vi "VisualizeBase.vi"() -> ()   [LabVIEW 2017, in "Visualization.lvlib" / "VisualizeBase_class.lvclass"]
uses:
  VisualizeBase_class.lvclass
  Framework/Bus_class/Bus.lvclass
  Typedefs/VisualizeData.ctl
  Typedefs/clVisualizeData.ctl
  Modules/EventPlugins/EventPluginBaseClass/TypeDefs/clEvtReportArray.ctl
  Modules/EventPlugins/EventPluginBaseClass/TypeDefs/clEvtReport.ctl
  Modules/EventPlugins/EventPluginBaseClass/TypeDefs/dblEvtSignalArray.ctl
  Modules/NetworkImpairmentModule/PublicAPI/Arguments/Broadcasts/dblNetworkTime.ctl
  Modules/NetworkImpairmentModule/PublicAPI/Arguments/Broadcasts/dblPktLoss.ctl
  Modules/FlagImpairModule/PublicAPI/Arguments/Broadcasts/ui32FlagImpairmentArray.ctl
  Framework/Bus_class/Broadcast/Typedefs/clDidInit.ctl
  QMH/Typedefs/clEvtRptArray.ctl
  QMH/Typedefs/clEvtRptSignal.ctl
  QMH/Typedefs/clPmuImpairRptArray.ctl
  QMH/Typedefs/clNetImpairmentTime.ctl
  QMH/Typedefs/clNetIPktLoss.ctl
  QMH/Typedefs/clFlagImpairArray.ctl
  Requests/clUserEventType.ctl
  <vilib>/event_ctls.llb/usereventprio.ctl
  <vilib>/Utility/miscctls.llb/LVStringsAndValuesArrayTypeDef_U8.ctl
  <vilib>/Utility/error.llb/Error Cluster From Error Code.vi
  <vilib>/ErrorRing/Error Ring.xnode
  <userlib>/NIST/NISTErrorLib/NISTErrorLib.lvlib
  Framework/Bus_class/Bus_class.lvlib
  Modules/EventModule/EventModule.lvlib
  Modules/PmuImpairModule/PmuImpairModule.lvlib
  Modules/NetworkImpairmentModule/NetworkImpairmentModule.lvlib
  Modules/FlagImpairModule/FlagImpairModule.lvlib
  Modules/EventPlugins/EventPluginBaseClass/EventPluginBaseClass.lvclass
  VisualizeApp_class/VisualizeAppBase_class.lvclass
panel:
  in  "QueName":string="BaseVisQue"
  in  "Bus Number":u8(ring) items=[""=0, "2"=2]
  out "ErrorArray":errorcluster[](array[cluster])
  in  "btnStop":bool
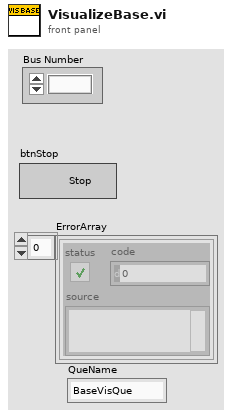
[diagram p1: front panel]
types:
  T1 = typedef "Visualization.lvlib/VisualizeBase_class.lvclass/VisualizeData.ctl" = T2[]
  T2 = typedef "Visualization.lvlib/VisualizeAppBase_class.lvclass/clVisualizeData.ctl" = cluster{"clEvtReportArray":T3, "dblEventSignalArray":T5, "clPmuImpairRptArray":T3, "dblNetworkTime":T6, "dblPktLoss":T7, "FlagImpairArray":T8, "TimeArray":dbl[]}
  T3 = typedef "EventPlugins.lvlib/EventPluginBaseClass.lvclass/clEvtReportArray.ctl" = T4[]
  T4 = typedef "EventPlugins.lvlib/EventPluginBaseClass.lvclass/clEvtReport.ctl" = cluster{"Timestamp":dbl, "Synx":cdb[], "Freq":dbl, "ROCOF":dbl, "ID":i16}
  T5 = typedef "EventPlugins.lvlib/EventPluginBaseClass.lvclass/dblEvtSignalArray.ctl" = dbl[][]
  T6 = typedef "NetworkImpairmentModule.lvlib/dblNetworkTime.ctl" = dbl[]
  T7 = typedef "NetworkImpairmentModule.lvlib/dblPktLoss.ctl" = dbl[]
  T8 = typedef "FlagImpairModule.lvlib/ui32FlagImpairmentArray.ctl" = u32[]
  T9 = typedef "Visualization.lvlib/VisualizeBase_class.lvclass/clRequestEvents.ctl" = cluster{"StopRequest":refnum<user-event>}
  T10 = typedef "Bus_class.lvlib/clBroadcastEvents.ctl" = cluster{"DidInit":refnum<user-event>, "DidStop":refnum<user-event>}
  T11 = typedef "EventModule.lvlib/clBroadcastEvents.ctl" = cluster{"DidInit":refnum<user-event>, "StatusUpdate":refnum<user-event>, "ErrorReport":refnum<user-event>, "DidStop":refnum<user-event>, "ReadEvtConfig":refnum<user-event>, "ReadTimeArray":refnum<user-event>, "ReadEvtParams":refnum<user-event>, "GetEvtReportArray":refnum<user-event>, "ReadPathToPlugin":refnum<user-event>, "GetEvtSignal":refnum<user-event>, "ReadBusNumber":refnum<user-event>}
  T12 = typedef "PmuImpairModule.lvlib/clBroadcastEvents.ctl" = cluster{"DidInit":refnum<user-event>, "StatusUpdate":refnum<user-event>, "ErrorReport":refnum<user-event>, "DidStop":refnum<user-event>, "ImpairConfig":refnum<user-event>, "ImpairParams":refnum<user-event>, "ImpairReports":refnum<user-event>, "PathToPlugin":refnum<user-event>, "BusNumber":refnum<user-event>}
  T13 = typedef "NetworkImpairmentModule.lvlib/clBroadcastEvents.ctl" = cluster{"DidInit":refnum<user-event>, "StatusUpdate":refnum<user-event>, "ErrorReport":refnum<user-event>, "DidStop":refnum<user-event>, "ReadNetImpParams":refnum<user-event>, "ReadLossThreshold":refnum<user-event>, "GetNetworkTime":refnum<user-event>, "GetPktLoss":refnum<user-event>, "ReadPathToPlugin":refnum<user-event>}
  T14 = typedef "FlagImpairModule.lvlib/clBroadcastEvents.ctl" = cluster{"DidInit":refnum<user-event>, "StatusUpdate":refnum<user-event>, "ErrorReport":refnum<user-event>, "DidStop":refnum<user-event>, "ReadFlagImpairConfig":refnum<user-event>, "ReadPluginINIFilePath":refnum<user-event>, "ReadFlagImpairParams":refnum<user-event>, "ReadTimeArray":refnum<user-event>, "GetFlagImpairment":refnum<user-event>}
  T15 = typedef "LVStringsAndValuesArrayTypeDef_U8.ctl" = cluster{"String":string, "Value":u8}[]
  T16 = typedef "Visualization.lvlib/VisualizeBase_class.lvclass/clEvtRptArray.ctl" = cluster{"BusIndex":i32, "clImpairReportArray":T3}
  T17 = typedef "Visualization.lvlib/VisualizeBase_class.lvclass/clPmuImpairRptArray.ctl" = cluster{"BusIndex":i32, "clImpairReportArray":T3}
  T18 = typedef "Visualization.lvlib/VisualizeBase_class.lvclass/clNetImpairmentTime.ctl" = cluster{"BusIndex":i32, "clNetImpairTimeArray":T6}
  T19 = typedef "Visualization.lvlib/VisualizeBase_class.lvclass/clNetIPktLoss.ctl" = cluster{"BusIndex":i32, "clNetPktLoss":T7}
  T20 = typedef "Visualization.lvlib/VisualizeBase_class.lvclass/clFlagImpairArray.ctl" = cluster{"BusIndex":i32, "FlagImpairArray":T8}
  T21 = typedef "Visualization.lvlib/VisualizeBase_class.lvclass/clEvtRptSignal.ctl" = cluster{"BusIndex":i32, "dblEventSignalArray":T5}
  T22 = typedef "Visualization.lvlib/VisualizeBase_class.lvclass/clUserEventType.ctl" = cluster{"BusIndex":i8, "Data":variant}
  T23 = typedef "usereventprio.ctl" = enum32{"high priority", "normal priority"}
  T24 = typedef "Bus_class.lvlib/clDidInit.ctl" = cluster{"Bus":refnum<vi>, "Init?":bool}
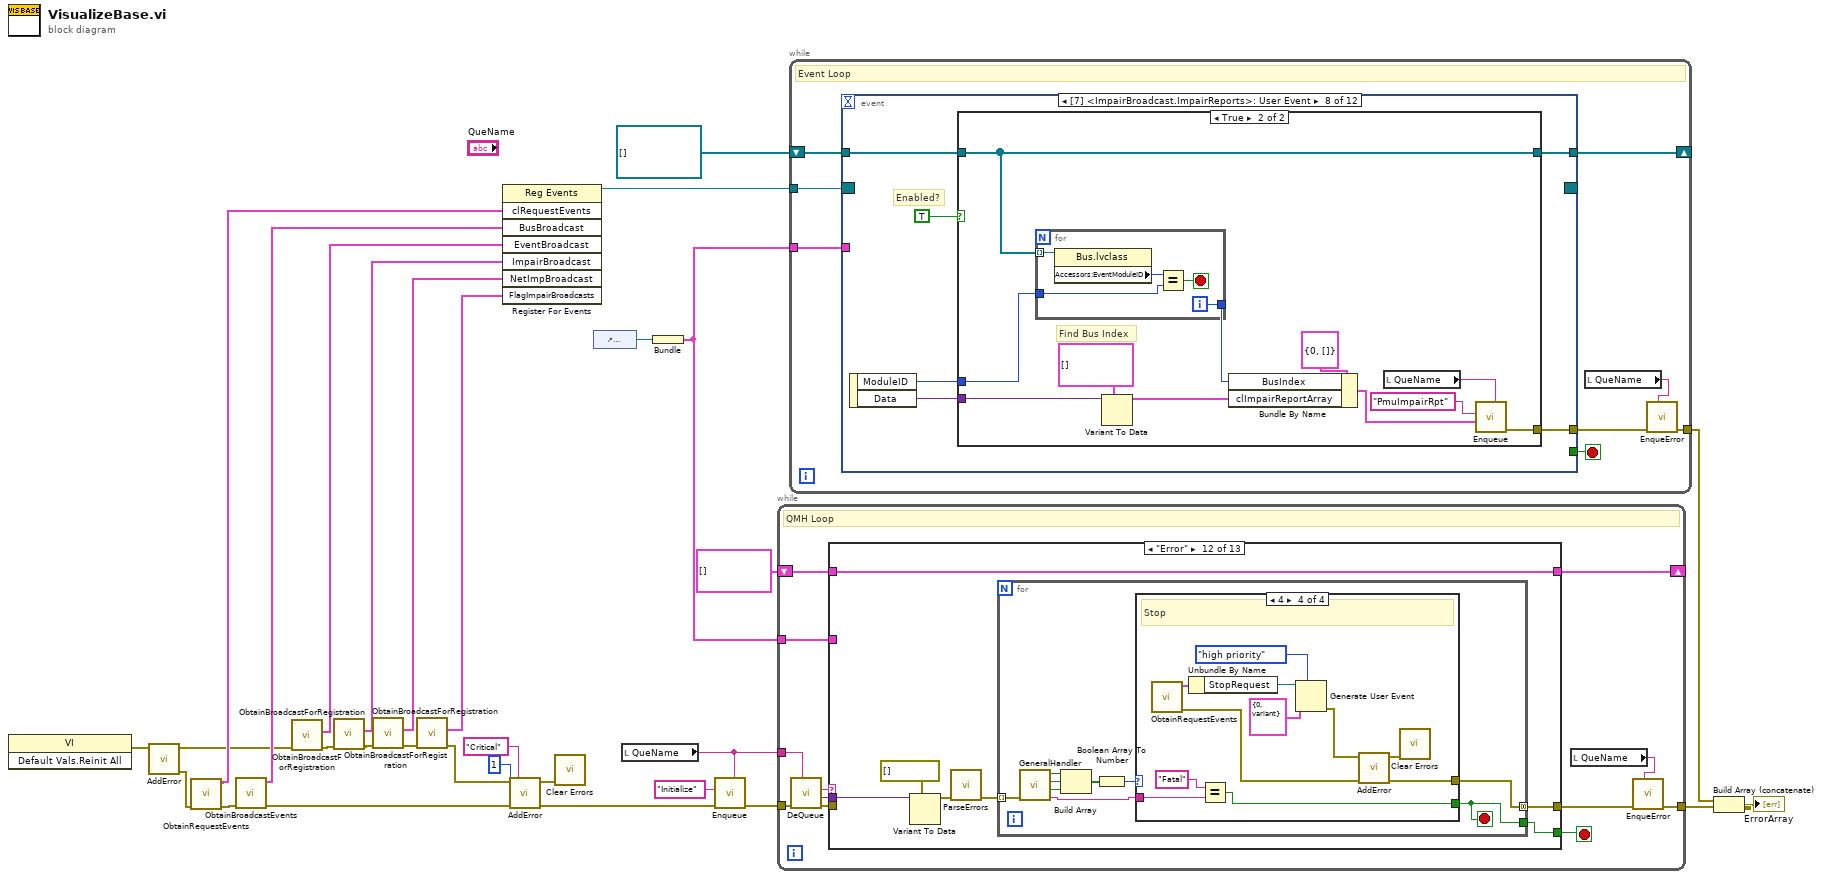
[diagram p0: block diagram]
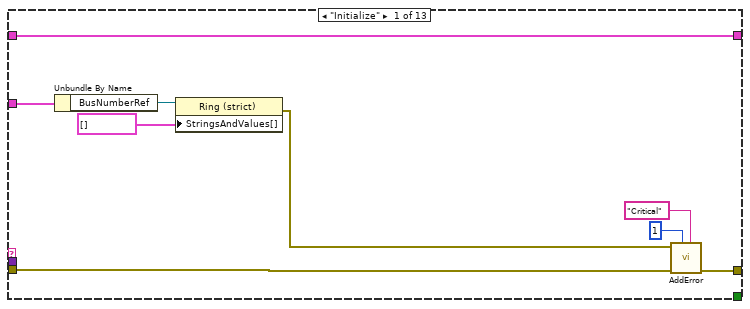
[diagram p2: hidden frame]
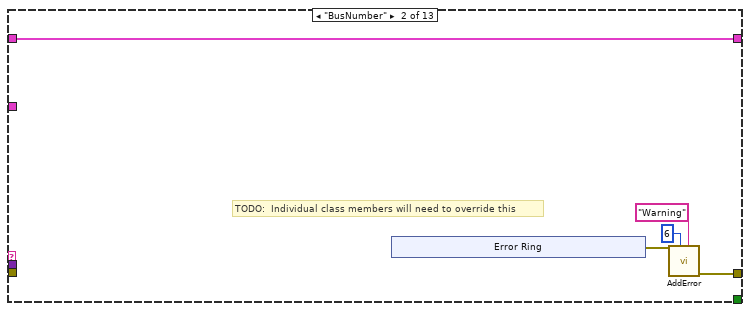
[diagram p3: hidden frame]
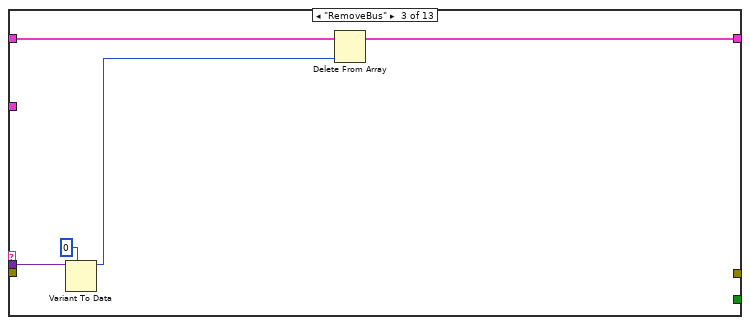
[diagram p4: hidden frame]
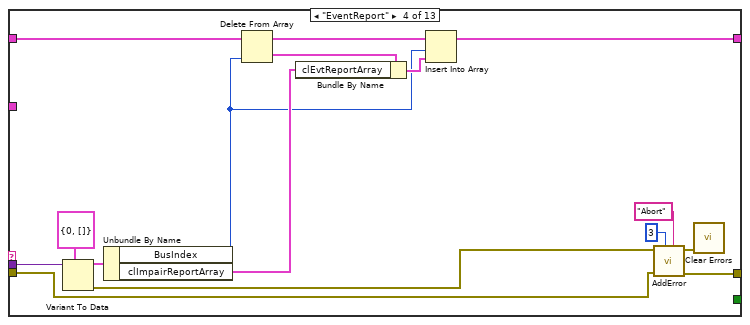
[diagram p5: hidden frame]
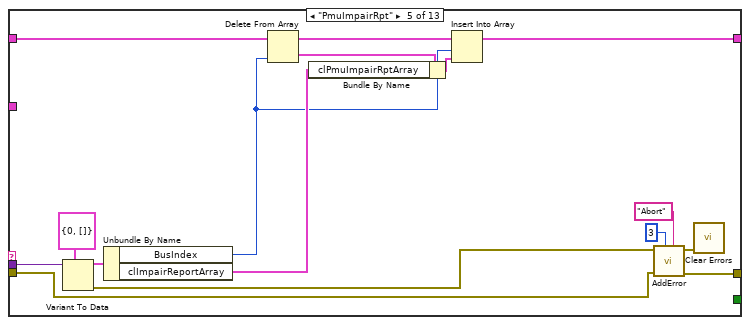
[diagram p6: hidden frame]
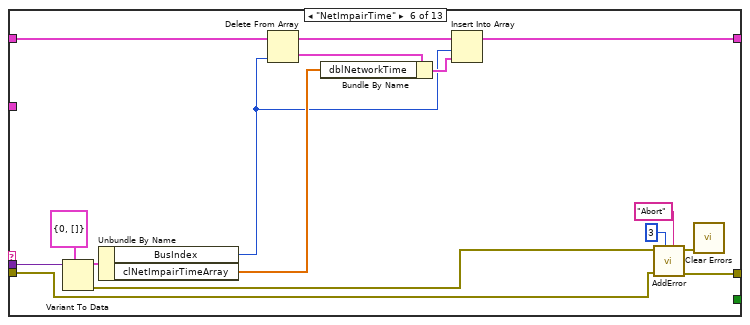
[diagram p7: hidden frame]
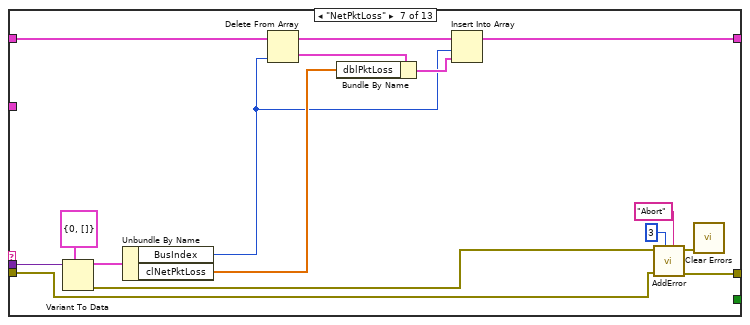
[diagram p8: hidden frame]
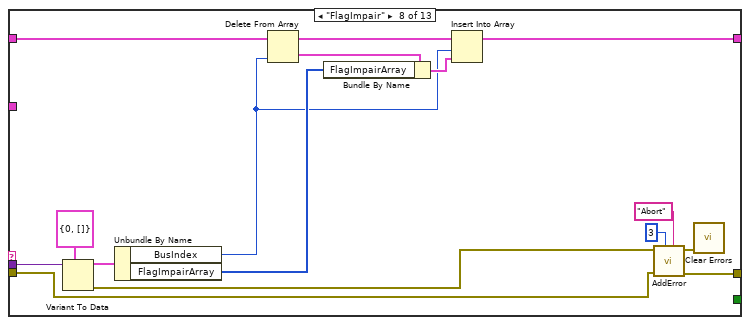
[diagram p9: hidden frame]
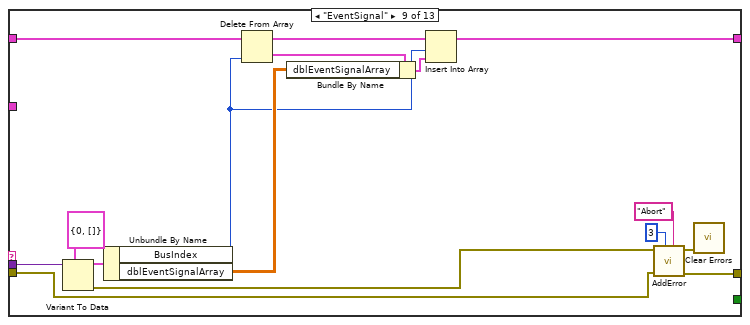
[diagram p10: hidden frame]
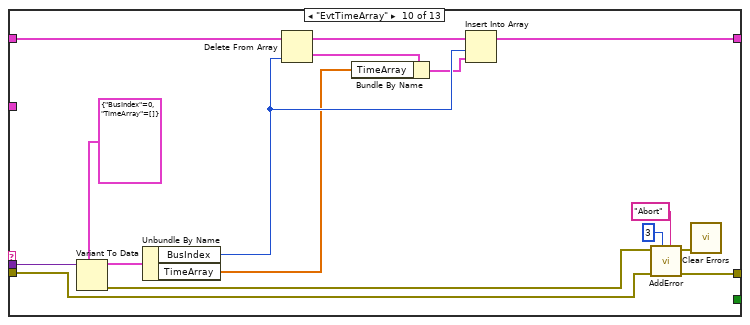
[diagram p11: hidden frame]
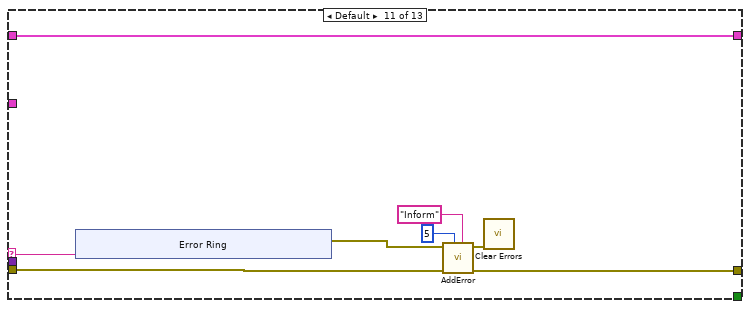
[diagram p12: hidden frame]
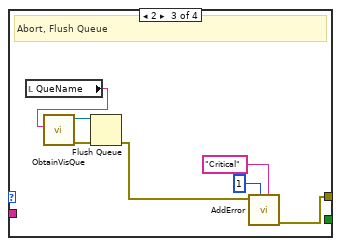
[diagram p15: hidden frame]
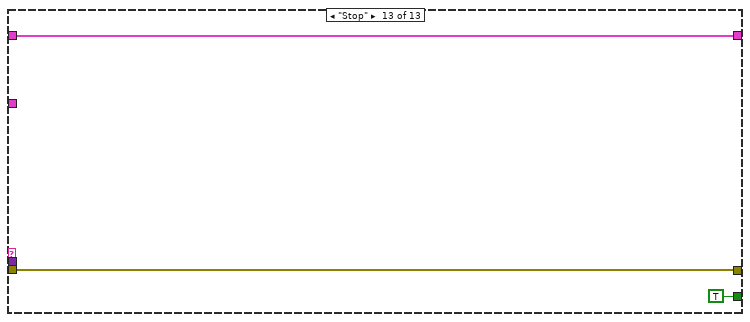
[diagram p16: hidden frame]
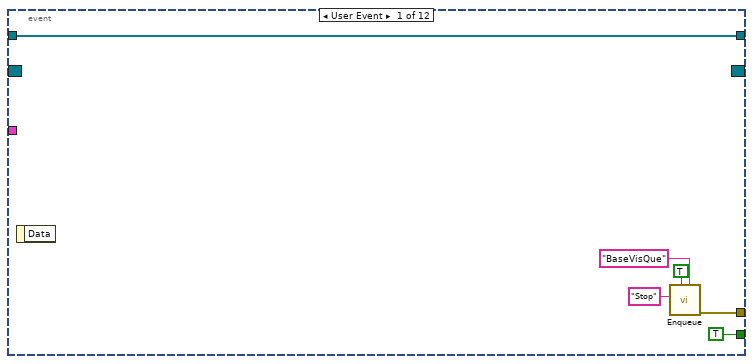
[diagram p17: hidden frame]
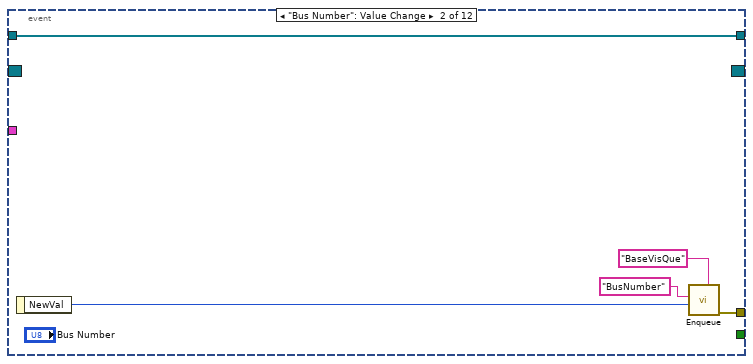
[diagram p18: hidden frame]
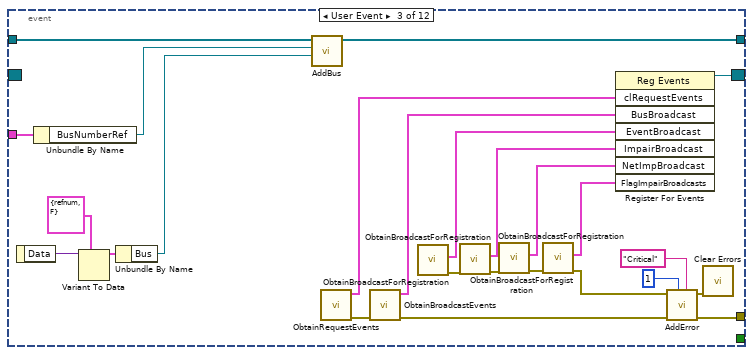
[diagram p19: hidden frame]
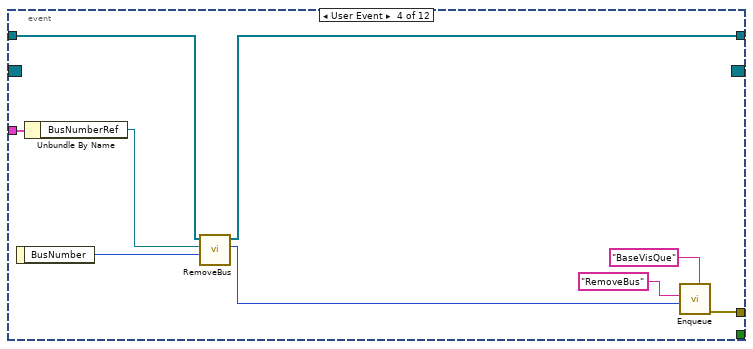
[diagram p20: hidden frame]
diagram:
  n1 = invoke class="VI" method="Default Vals.Reinit All"() -> (error out=w19:errorcluster)  [unwired: 3 in, 2 out]
  n2 = call <userlib>:"AddError.vi"("error in (no error)"=w19) -> ("ErrorArray"=w18:errorcluster[], "error out"=w10:errorcluster)  [unwired: 9 in]
  n3 = call "ObtainRequestEvents.vi"("Error"=w18) -> ("Error"=w23:errorcluster[], "clRequestEvents"=w28:T9)  [unwired: 9 in]
  n4 = call "ObtainBroadcastEvents.vi"("ErrorArray"=w23) -> ("ErrorArray"=w9:errorcluster[], "BusBroadcast"=w22:T10)  [unwired: 9 in]
  n5 = call "ObtainBroadcastForRegistration.vi"("error in (no error)"=w10) -> ("error out"=w13:errorcluster, "EventBroadcast"=w17:T11)  [unwired: 9 in]
  n6 = call "ObtainBroadcastForRegistration.vi"("error in (no error)"=w13) -> ("error out"=w12:errorcluster, "ImpairBroadcast"=w16:T12)  [unwired: 9 in]
  n7 = call "ObtainBroadcastForRegistration.vi"("error in (no error)"=w12) -> ("error out"=w11:errorcluster, "NetImpBroadcast"=w15:T13)  [unwired: 9 in]
  n8 = call "ObtainBroadcastForRegistration.vi"("error in (no error)"=w11) -> ("error out"=w8:errorcluster, "FlagImpairBroadcasts"=w14:T14)  [unwired: 9 in]
  n9 = register-events(w28, w22, w17, w16, w15, w14) -> (reference out=w27:refnum<event-registration>)  [unwired: 2 in, 1 out]
  n10 = call <userlib>:"AddError.vi"("Severity"="Critical" ("String"), "Priority"=u8 1, "ErrorArray"=w9, "error in (no error)"=w8) -> ("ErrorArray"=w5:errorcluster[], "error out"=w2:errorcluster)  [unwired: 6 in]
  n11 = call <vilib>:"Clear Errors.vi"("error in (no error)"=w2) -> ()  [unwired: 5 in, 2 out]
  n12 = control-ref of="BusNumberRef"() -> (w21:refnum<vi>)
  n13 = local read "QueName"() -> (w1:string)
  n14 = Bundle("BusNumberRef"=w21) -> (w3:cluster{"BusNumberRef":refnum<vi>})  [unwired: 1 in]
  n15 = call "Enqueue.vi"("QueName"=w1, "Error"=w5, "Message"="Initialize") -> ("Error"=w29:errorcluster[])  [unwired: 8 in]
  n16 = while {
    tunnel: w29 -> [w42]
    tunnel: [w36] -> w26
    tunnel: w3 -> [w35]
    shift-right: [w33] -> _
    shift-left: T1 [] ("VisualizeData") -> [w34]
    tunnel: w1 -> [w31]
    stop <- w37 stop-if-true
    # "QMH Loop"
    n17 = call "DeQueue.vi"("QueName"=w31, "Error"=w42) -> ("Error"=w39:errorcluster[], "Data"=w40:variant, "Message"=w41:string)  [unwired: 7 in]
    n18 = case shown="\"Error\"" w41 {
      selector: w41 -> [_ _ _ _ _ _ _ _ _ _ w186 _ _]
      tunnel: w40 -> [_ _ w66 w82 w98 w114 w130 w146 w162 w169 _ w200 _]
      tunnel: w39 -> [w48 _ _ w67 w83 w99 w115 w131 w147 w163 w184 _ w229]
      tunnel: [w47 w56 _ w72 w88 w104 w120 w136 w152 w165 w183 w196 w229] -> w38
      tunnel: [_ _ _ _ _ _ _ _ _ _ _ w195 TRUE] -> w37
      tunnel: w35 -> [w51 _ _ _ _ _ _ _ _ _ _ _ _]
      tunnel: w34 -> [w43 w52 w64 w78 w94 w110 w126 w142 w158 w171 w179 w194 w228]
      tunnel: [w43 w52 w63 w79 w95 w111 w127 w143 w159 w170 w179 w194 w228] -> w33
      frame "Initialize" {
        n19 = Unbundle By Name(w51) -> ("BusNumberRef"=w50:refnum<vi>)
        n20 = property class="Ring (strict)"(reference=w50, "StringsAndValues[]"=T15 [] ("Strings And Values []")) -> (error out=w46:errorcluster)  [unwired: 1 in, 1 out]
        n21 = call <userlib>:"AddError.vi"("Severity"="Critical" ("String"), "Priority"=u8 1, "ErrorArray"=w48, "error in (no error)"=w46) -> ("ErrorArray"=w47:errorcluster[])  [unwired: 6 in, 1 out]
      }
      frame "BusNumber" {
        # "TODO:  Individual class members will need to override this"
        n22 = xnode "Error Ring"() -> ("error out"=w55:errorcluster)
        n23 = call <userlib>:"AddError.vi"("Severity"="Warning" ("String"), "Priority"=u8 6, "error in (no error)"=w55) -> ("ErrorArray"=w56:errorcluster[])  [unwired: 7 in, 1 out]
      }
      frame "RemoveBus" {
        n24 = Variant To Data(type=0, Variant=w66) -> (data=w62:i32)  [unwired: 1 in, 1 out]
        n25 = Delete From Array(array=w64, index=w62) -> (array with subset deleted=w63:T1)  [unwired: 1 in, 1 out]
      }
      frame "EventReport" {
        n26 = Variant To Data(type=T16 {"BusIndex"=0, "clImpairReportArray"=[]} ("clEvtReportArray"), Variant=w82) -> (data=w80:T16, error out=w71:errorcluster)  [unwired: 1 in]
        n27 = Unbundle By Name(w80) -> ("BusIndex"=w73:i32, "clImpairReportArray"=w75:T3)
        n28 = Delete From Array(array=w78, index=w73) -> (deleted portion=w76:T2, array with subset deleted=w77:T1)  [unwired: 1 in]
        n29 = Bundle By Name(cluster=w76, "clEvtReportArray"=w75) -> (w74:T2)
        n30 = Insert Into Array(array=w77, index=w73, new element=w74) -> (w79:T1)
        n31 = call <userlib>:"AddError.vi"("Severity"="Abort" ("String"), "Priority"=u8 3, "ErrorArray"=w67, "error in (no error)"=w71) -> ("ErrorArray"=w72:errorcluster[], "error out"=w70:errorcluster)  [unwired: 6 in]
        n32 = call <vilib>:"Clear Errors.vi"("error in (no error)"=w70) -> ()  [unwired: 5 in, 2 out]
      }
      frame "PmuImpairRpt" {
        n33 = Variant To Data(type=T17 {"BusIndex"=0, "clImpairReportArray"=[]} ("clImpairReportArray"), Variant=w98) -> (data=w96:T17, error out=w87:errorcluster)  [unwired: 1 in]
        n34 = Unbundle By Name(w96) -> ("BusIndex"=w89:i32, "clImpairReportArray"=w91:T3)
        n35 = Delete From Array(array=w94, index=w89) -> (deleted portion=w92:T2, array with subset deleted=w93:T1)  [unwired: 1 in]
        n36 = Bundle By Name(cluster=w92, "clPmuImpairRptArray"=w91) -> (w90:T2)
        n37 = Insert Into Array(array=w93, index=w89, new element=w90) -> (w95:T1)
        n38 = call <userlib>:"AddError.vi"("Severity"="Abort" ("String"), "Priority"=u8 3, "ErrorArray"=w83, "error in (no error)"=w87) -> ("ErrorArray"=w88:errorcluster[], "error out"=w86:errorcluster)  [unwired: 6 in]
        n39 = call <vilib>:"Clear Errors.vi"("error in (no error)"=w86) -> ()  [unwired: 5 in, 2 out]
      }
      frame "NetImpairTime" {
        n40 = Variant To Data(type=T18 {"BusIndex"=0, "clNetImpairTimeArray"=[]} ("clImpairReportArray"), Variant=w114) -> (data=w112:T18, error out=w103:errorcluster)  [unwired: 1 in]
        n41 = Unbundle By Name(w112) -> ("BusIndex"=w105:i32, "clNetImpairTimeArray"=w107:T6)
        n42 = Delete From Array(array=w110, index=w105) -> (deleted portion=w108:T2, array with subset deleted=w109:T1)  [unwired: 1 in]
        n43 = Bundle By Name(cluster=w108, "dblNetworkTime"=w107) -> (w106:T2)
        n44 = Insert Into Array(array=w109, index=w105, new element=w106) -> (w111:T1)
        n45 = call <userlib>:"AddError.vi"("Severity"="Abort" ("String"), "Priority"=u8 3, "ErrorArray"=w99, "error in (no error)"=w103) -> ("ErrorArray"=w104:errorcluster[], "error out"=w102:errorcluster)  [unwired: 6 in]
        n46 = call <vilib>:"Clear Errors.vi"("error in (no error)"=w102) -> ()  [unwired: 5 in, 2 out]
      }
      frame "NetPktLoss" {
        n47 = Variant To Data(type=T19 {"BusIndex"=0, "clNetPktLoss"=[]} ("clNetPktLoss"), Variant=w130) -> (data=w128:T19, error out=w119:errorcluster)  [unwired: 1 in]
        n48 = Unbundle By Name(w128) -> ("BusIndex"=w121:i32, "clNetPktLoss"=w123:T7)
        n49 = Delete From Array(array=w126, index=w121) -> (deleted portion=w124:T2, array with subset deleted=w125:T1)  [unwired: 1 in]
        n50 = Bundle By Name(cluster=w124, "dblPktLoss"=w123) -> (w122:T2)
        n51 = Insert Into Array(array=w125, index=w121, new element=w122) -> (w127:T1)
        n52 = call <userlib>:"AddError.vi"("Severity"="Abort" ("String"), "Priority"=u8 3, "ErrorArray"=w115, "error in (no error)"=w119) -> ("ErrorArray"=w120:errorcluster[], "error out"=w118:errorcluster)  [unwired: 6 in]
        n53 = call <vilib>:"Clear Errors.vi"("error in (no error)"=w118) -> ()  [unwired: 5 in, 2 out]
      }
      frame "FlagImpair" {
        n54 = Variant To Data(type=T20 {"BusIndex"=0, "FlagImpairArray"=[]} ("clFlagImpairArray"), Variant=w146) -> (data=w144:T20, error out=w135:errorcluster)  [unwired: 1 in]
        n55 = Unbundle By Name(w144) -> ("BusIndex"=w137:i32, "FlagImpairArray"=w139:T8)
        n56 = Delete From Array(array=w142, index=w137) -> (deleted portion=w140:T2, array with subset deleted=w141:T1)  [unwired: 1 in]
        n57 = Bundle By Name(cluster=w140, "FlagImpairArray"=w139) -> (w138:T2)
        n58 = Insert Into Array(array=w141, index=w137, new element=w138) -> (w143:T1)
        n59 = call <userlib>:"AddError.vi"("Severity"="Abort" ("String"), "Priority"=u8 3, "ErrorArray"=w131, "error in (no error)"=w135) -> ("ErrorArray"=w136:errorcluster[], "error out"=w134:errorcluster)  [unwired: 6 in]
        n60 = call <vilib>:"Clear Errors.vi"("error in (no error)"=w134) -> ()  [unwired: 5 in, 2 out]
      }
      frame "EventSignal" {
        n61 = Variant To Data(type=T21 {"BusIndex"=0, "dblEventSignalArray"=[]} ("clEvtReportArray"), Variant=w162) -> (data=w160:T21, error out=w151:errorcluster)  [unwired: 1 in]
        n62 = Unbundle By Name(w160) -> ("BusIndex"=w153:i32, "dblEventSignalArray"=w155:T5)
        n63 = Delete From Array(array=w158, index=w153) -> (deleted portion=w156:T2, array with subset deleted=w157:T1)  [unwired: 1 in]
        n64 = Bundle By Name(cluster=w156, "dblEventSignalArray"=w155) -> (w154:T2)
        n65 = Insert Into Array(array=w157, index=w153, new element=w154) -> (w159:T1)
        n66 = call <userlib>:"AddError.vi"("Severity"="Abort" ("String"), "Priority"=u8 3, "ErrorArray"=w147, "error in (no error)"=w151) -> ("ErrorArray"=w152:errorcluster[], "error out"=w150:errorcluster)  [unwired: 6 in]
        n67 = call <vilib>:"Clear Errors.vi"("error in (no error)"=w150) -> ()  [unwired: 5 in, 2 out]
      }
      frame "EvtTimeArray" {
        n68 = Variant To Data(type=cluster{"BusIndex":i32, "TimeArray":dbl[]} {"BusIndex"=0, "TimeArray"=[]} ("cluster"), Variant=w169) -> (data=w172:cluster{"BusIndex":i32, "TimeArray":dbl[]}, error out=w164:errorcluster)  [unwired: 1 in]
        n69 = Unbundle By Name(w172) -> ("BusIndex"=w177:i32, "TimeArray"=w175:dbl[])
        n70 = Delete From Array(array=w171, index=w177) -> (deleted portion=w174:T2, array with subset deleted=w173:T1)  [unwired: 1 in]
        n71 = Bundle By Name(cluster=w174, "TimeArray"=w175) -> (w176:T2)
        n72 = Insert Into Array(array=w173, index=w177, new element=w176) -> (w170:T1)
        n73 = call <userlib>:"AddError.vi"("Severity"="Abort" ("String"), "Priority"=u8 3, "ErrorArray"=w163, "error in (no error)"=w164) -> ("ErrorArray"=w165:errorcluster[], "error out"=w166:errorcluster)  [unwired: 6 in]
        n74 = call <vilib>:"Clear Errors.vi"("error in (no error)"=w166) -> ()  [unwired: 5 in, 2 out]
      }
      frame Default {
        n75 = xnode "Error Ring"("parameter 0"=w186) -> ("error out"=w185:errorcluster)
        n76 = call <userlib>:"AddError.vi"("Severity"="Inform" ("String"), "Priority"=u8 5, "ErrorArray"=w184, "error in (no error)"=w185) -> ("ErrorArray"=w183:errorcluster[], "error out"=w182:errorcluster)  [unwired: 6 in]
        n77 = call <vilib>:"Clear Errors.vi"("error in (no error)"=w182) -> ()  [unwired: 5 in, 2 out]
      }
      frame "Error" {
        n78 = Variant To Data(type=errorcluster[] [], Variant=w200) -> (data=w198:errorcluster[])  [unwired: 1 in, 1 out]
        n79 = call <userlib>:"ParseErrors.vi"("ErrorArray"=w198) -> ("ErrorArray"=w197:errorcluster[])  [unwired: 8 in, 2 out]
        n80 = for {
          tunnel: w197 -> [w209] mode=indexing
          tunnel: [w203] -> w196 mode=concatenating
          tunnel: [w201] -> w195
          stop <- w201 stop-if-true
          n81 = call <userlib>:"GeneralHandler.vi"("error in (no error)"=w209) -> ("Severity"=w202:string, "Stop"=w206:bool, "Abort"=w207:bool, "Continue"=w208:bool)  [unwired: 7 in]
          n82 = Build Array(w208, w207, w206) -> (w205:bool[])
          n83 = Boolean Array To Number(Boolean array=w205) -> (number=w204:u32)
          n84 = case shown="4" w204 {
            tunnel: [_ _ w214 w225] -> w203
            tunnel: w202 -> [_ _ _ w219]
            tunnel: [_ _ _ w217] -> w201
            frame 0, Default {
              # "No Dialog"
            }
            frame 1 {
              # "Continue"
            }
            frame 2 {
              # "Abort, Flush Queue"
              n85 = local read "QueName"() -> (w210:string)
              n86 = call "ObtainVisQue.vi"("QueName"=w210) -> ("error out"=w216:errorcluster, "queue out"=w215:refnum<queue>)  [unwired: 9 in]
              n87 = Flush Queue(queue=w215, error in (no error)=w216) -> (error out=w213:errorcluster)  [unwired: 2 out]
              n88 = call <userlib>:"AddError.vi"("Severity"="Critical" ("String"), "Priority"=u8 1, "error in (no error)"=w213) -> ("ErrorArray"=w214:errorcluster[])  [unwired: 7 in, 1 out]
            }
            frame 4 {
              # "Stop"
              n89 = call "ObtainRequestEvents.vi"() -> ("Error"=w223:errorcluster[], "clRequestEvents"=w227:T9)  [unwired: 10 in]
              n90 = Unbundle By Name(w227) -> ("StopRequest"=w226:refnum<user-event>)
              n91 = Equal?(x="Fatal", y=w219) -> (x = y?=w217:bool)
              n92 = Generate User Event(priority (normal)=usereventprio."high priority", user event=w226, event data cluster=T22 {"BusIndex"=0, "Data"=variant} ("event data")) -> (error out=w224:errorcluster)  [unwired: 1 in, 1 out]
              n93 = call <userlib>:"AddError.vi"("ErrorArray"=w223, "error in (no error)"=w224) -> ("ErrorArray"=w225:errorcluster[], "error out"=w220:errorcluster)  [unwired: 8 in]
              n94 = call <vilib>:"Clear Errors.vi"("error in (no error)"=w220) -> ()  [unwired: 5 in, 2 out]
            }
          }
        }
      }
      frame "Stop" {
      }
    }
    n95 = local read "QueName"() -> (w32:string)
    n96 = call "EnqueError.vi"("QueName"=w32, "Error"=w38) -> ("Error"=w36:errorcluster[])  [unwired: 9 in]
  }
  n97 = while {
    tunnel: w27 -> [w238]
    tunnel: [w235] -> w25
    tunnel: w3 -> [w234]
    shift-right: [w232] -> _
    shift-left: refnum<class "Bus.lvclass">[] [] -> [w233]
    stop <- w237 stop-if-true
    # "Event Loop"
    n98 = event shown="[7] <ImpairBroadcast.ImpairReports>: User Event" {
      selector: w238 -> [_ _ _ _ _ _ _ _ _ _ _ _]
      dyn-events: [_ _ w258 _ _ _ _ _ _ _ _ _] -> _
      timeout: _ -> [_ _ _ _ _ _ _ _ _ _ _ _]
      tunnel: [TRUE _ _ _ _ _ _ _ _ _ _ _] -> w237
      tunnel: [w243 w249 w261 w279 w285 w314 w337 w360 w383 w406 w429 w456] -> w236
      tunnel: w234 -> [_ _ w271 w283 _ _ _ _ _ _ _ _]
      tunnel: w233 -> [w240 w246 w270 w282 w286 w317 w340 w363 w386 w409 w432 w450]
      tunnel: [w240 w246 w267 w281 w284 w312 w335 w358 w381 w404 w427 w450] -> w232
      event User Event {
        n99 = event-data() -> ()  [unwired: 1 in, 1 out]
        n100 = call "Enqueue.vi"("QueName"="BaseVisQue", "Priority? (F)"=TRUE, "Message"="Stop") -> ("Error"=w243:errorcluster[])  [unwired: 8 in]
      }
      event "Bus Number": Value Change {
        n101 = event-data() -> ("NewVal"=w248:u8)  [unwired: 1 in]
        n102 = call "Enqueue.vi"("QueName"="BaseVisQue", "Data"=w248, "Message"="BusNumber") -> ("Error"=w249:errorcluster[])  [unwired: 8 in]
      }
      event User Event {
        n103 = event-data() -> ("Data"=w274:variant)  [unwired: 1 in]
        n104 = Unbundle By Name(w271) -> ("BusNumberRef"=w269:refnum<vi>)
        n105 = Variant To Data(type=T24 {"Bus"=refnum, "Init?"=FALSE} ("clBusDidInit"), Variant=w274) -> (data=w272:T24)  [unwired: 1 in, 1 out]
        n106 = Unbundle By Name(w272) -> ("Bus"=w268:refnum<vi>)
        n107 = call "AddBus.vi"("BusRef"=w268, "BusNumberRef"=w269, "BusArray"=w270) -> ("BusArray"=w267:refnum<class "Bus.lvclass">[])  [unwired: 8 in]
        n108 = call "ObtainRequestEvents.vi"() -> ("Error"=w253:errorcluster[], "clRequestEvents"=w251:T9)  [unwired: 10 in]
        n109 = call "ObtainBroadcastEvents.vi"("ErrorArray"=w253) -> ("ErrorArray"=w252:errorcluster[], "BusBroadcast"=w250:T10)  [unwired: 9 in]
        n110 = call "ObtainBroadcastForRegistration.vi"() -> ("error out"=w266:errorcluster, "EventBroadcast"=w257:T11)  [unwired: 10 in]
        n111 = call "ObtainBroadcastForRegistration.vi"("error in (no error)"=w266) -> ("error out"=w265:errorcluster, "ImpairBroadcast"=w256:T12)  [unwired: 9 in]
        n112 = call "ObtainBroadcastForRegistration.vi"("error in (no error)"=w265) -> ("error out"=w264:errorcluster, "NetImpBroadcast"=w255:T13)  [unwired: 9 in]
        n113 = call "ObtainBroadcastForRegistration.vi"("error in (no error)"=w264) -> ("error out"=w259:errorcluster, "FlagImpairBroadcasts"=w254:T14)  [unwired: 9 in]
        n114 = register-events(w251, w250, w257, w256, w255, w254) -> (reference out=w258:refnum<event-registration>)  [unwired: 2 in, 1 out]
        n115 = call <userlib>:"AddError.vi"("Severity"="Critical" ("String"), "Priority"=u8 1, "ErrorArray"=w252, "error in (no error)"=w259) -> ("ErrorArray"=w261:errorcluster[], "error out"=w260:errorcluster)  [unwired: 6 in]
        n116 = call <vilib>:"Clear Errors.vi"("error in (no error)"=w260) -> ()  [unwired: 5 in, 2 out]
      }
      event User Event {
        n117 = event-data() -> ("BusNumber"=w276:i8)  [unwired: 1 in]
        n118 = Unbundle By Name(w283) -> ("BusNumberRef"=w280:refnum<vi>)
        n119 = call "RemoveBus.vi"("BusArray"=w282, "BusNumberRef"=w280, "BusNumber"=w276) -> ("BusArray"=w281:refnum<class "Bus.lvclass">[], "BusIndex"=w278:i32)  [unwired: 6 in]
        n120 = call "Enqueue.vi"("QueName"="BaseVisQue", "Data"=w278, "Message"="RemoveBus") -> ("Error"=w279:errorcluster[])  [unwired: 8 in]
      }
      event User Event {
        w287 = TRUE  # Enabled?
        n121 = event-data() -> ("ModuleID"=w289:i32, "Data"=w288:variant)  [unwired: 1 in]
        n122 = case shown="True" w287 {
          tunnel: [w290 w306] -> w284
          tunnel: w286 -> [w290 w306]
          tunnel: w289 -> [_ w303]
          tunnel: w288 -> [_ w305]
          tunnel: [_ w293] -> w285
          frame False {
          }
          frame True {
            n123 = Variant To Data(type=dbl[] [], Variant=w305) -> (data=w302:dbl[], error out=w298:errorcluster)  [unwired: 1 in]
            n124 = for {
              tunnel: w306 -> [w311] mode=indexing
              tunnel: w303 -> [w309]
              tunnel: [w307] -> w292
              i -> [w307]
              stop <- w308 stop-if-true
              # "Find Bus Index"
              n125 = property class="Bus.lvclass"(reference=w311) -> ("Accessors:EventModuleID"=w310:i32)  [unwired: 1 in, 2 out]
              n126 = Equal?(x=w310, y=w309) -> (x = y?=w308:bool)
            }
            n127 = call <userlib>:"AddError.vi"("Severity"="Critical" ("String"), "Priority"=u8 1, "error in (no error)"=w298) -> ("ErrorArray"=w294:errorcluster[], "error out"=w297:errorcluster)  [unwired: 7 in]
            n128 = call <vilib>:"Clear Errors.vi"("error in (no error)"=w297) -> ()  [unwired: 5 in, 2 out]
            n129 = Bundle(w292, w302) -> (w301:cluster{i32, dbl[]})  [unwired: 1 in]
            n130 = To Variant(anything=w301) -> (Variant=w300:variant)
            n131 = call "Enqueue.vi"("QueName"="BaseVisQue", "Error"=w294, "Data"=w300, "Message"="EvtTimeArray") -> ("Error"=w293:errorcluster[])  [unwired: 7 in]
          }
        }
      }
      event User Event {
        # "Enabled?"
        n132 = event-data() -> ("ModuleID"=w316:i32, "Data"=w315:variant)  [unwired: 1 in]
        n133 = case shown="True" TRUE {
          tunnel: w317 -> [w318 w320]
          tunnel: w316 -> [_ w329]
          tunnel: w315 -> [_ w327]
          tunnel: [_ w324] -> w314
          tunnel: [w318 w320] -> w312
          frame False {
          }
          frame True {
            # "Find Bus Index"
            n134 = for {
              tunnel: w320 -> [w334] mode=indexing
              tunnel: w329 -> [w332]
              tunnel: [w330] -> w328
              i -> [w330]
              stop <- w331 stop-if-true
              n135 = property class="Bus.lvclass"(reference=w334) -> ("Accessors:EventModuleID"=w333:i32)  [unwired: 1 in, 2 out]
              n136 = Equal?(x=w333, y=w332) -> (x = y?=w331:bool)
            }
            n137 = Variant To Data(type=T3 [] ("clEvtReportArray"), Variant=w327) -> (data=w325:T3)  [unwired: 1 in, 1 out]
            n138 = Bundle By Name(cluster=T16 {"BusIndex"=0, "clImpairReportArray"=[]} ("clEvtReportArray"), "BusIndex"=w328, "clImpairReportArray"=w325) -> (w323:T16)
            n139 = local read "QueName"() -> (w319:string)
            n140 = call "Enqueue.vi"("QueName"=w319, "Data"=w323, "Message"="EventReport") -> ("Error"=w324:errorcluster[])  [unwired: 8 in]
          }
        }
      }
      event User Event {
        # "Enabled?"
        n141 = event-data() -> ("ModuleID"=w339:i32, "Data"=w338:variant)  [unwired: 1 in]
        n142 = case shown="True" TRUE {
          tunnel: w340 -> [w341 w343]
          tunnel: w339 -> [_ w352]
          tunnel: w338 -> [_ w350]
          tunnel: [_ w347] -> w337
          tunnel: [w341 w343] -> w335
          frame False {
          }
          frame True {
            # "Find Bus Index"
            n143 = for {
              tunnel: w343 -> [w357] mode=indexing
              tunnel: w352 -> [w355]
              tunnel: [w353] -> w351
              i -> [w353]
              stop <- w354 stop-if-true
              n144 = property class="Bus.lvclass"(reference=w357) -> ("Accessors:EventModuleID"=w356:i32)  [unwired: 1 in, 2 out]
              n145 = Equal?(x=w356, y=w355) -> (x = y?=w354:bool)
            }
            n146 = Variant To Data(type=T5 [] ("dblEventSignalArray"), Variant=w350) -> (data=w348:T5)  [unwired: 1 in, 1 out]
            n147 = Bundle By Name(cluster=T21 {"BusIndex"=0, "dblEventSignalArray"=[]} ("clEvtReportArray"), "BusIndex"=w351, "dblEventSignalArray"=w348) -> (w346:T21)
            n148 = local read "QueName"() -> (w342:string)
            n149 = call "Enqueue.vi"("QueName"=w342, "Data"=w346, "Message"="EventSignal") -> ("Error"=w347:errorcluster[])  [unwired: 8 in]
          }
        }
      }
      event User Event {
        # "Enabled?"
        n150 = event-data() -> ("ModuleID"=w362:i32, "Data"=w361:variant)  [unwired: 1 in]
        n151 = case shown="True" TRUE {
          tunnel: w363 -> [w364 w366]
          tunnel: w362 -> [_ w375]
          tunnel: w361 -> [_ w373]
          tunnel: [_ w370] -> w360
          tunnel: [w364 w366] -> w358
          frame False {
          }
          frame True {
            # "Find Bus Index"
            n152 = for {
              tunnel: w366 -> [w380] mode=indexing
              tunnel: w375 -> [w378]
              tunnel: [w376] -> w374
              i -> [w376]
              stop <- w377 stop-if-true
              n153 = property class="Bus.lvclass"(reference=w380) -> ("Accessors:EventModuleID"=w379:i32)  [unwired: 1 in, 2 out]
              n154 = Equal?(x=w379, y=w378) -> (x = y?=w377:bool)
            }
            n155 = Variant To Data(type=T3 [] ("clEvtReportArray"), Variant=w373) -> (data=w371:T3)  [unwired: 1 in, 1 out]
            n156 = Bundle By Name(cluster=T17 {"BusIndex"=0, "clImpairReportArray"=[]} ("clEvtReportArray"), "BusIndex"=w374, "clImpairReportArray"=w371) -> (w369:T17)
            n157 = local read "QueName"() -> (w365:string)
            n158 = call "Enqueue.vi"("QueName"=w365, "Data"=w369, "Message"="PmuImpairRpt") -> ("Error"=w370:errorcluster[])  [unwired: 8 in]
          }
        }
      }
      event User Event {
        # "Enabled?"
        n159 = event-data() -> ("ModuleID"=w385:i32, "Data"=w384:variant)  [unwired: 1 in]
        n160 = case shown="True" TRUE {
          tunnel: w386 -> [w387 w389]
          tunnel: w385 -> [_ w398]
          tunnel: w384 -> [_ w396]
          tunnel: [_ w393] -> w383
          tunnel: [w387 w389] -> w381
          frame False {
          }
          frame True {
            # "Find Bus Index"
            n161 = for {
              tunnel: w389 -> [w403] mode=indexing
              tunnel: w398 -> [w401]
              tunnel: [w399] -> w397
              i -> [w399]
              stop <- w400 stop-if-true
              n162 = property class="Bus.lvclass"(reference=w403) -> ("Accessors:EventModuleID"=w402:i32)  [unwired: 1 in, 2 out]
              n163 = Equal?(x=w402, y=w401) -> (x = y?=w400:bool)
            }
            n164 = Variant To Data(type=T6 [] ("dblNetworkTime"), Variant=w396) -> (data=w394:T6)  [unwired: 1 in, 1 out]
            n165 = Bundle By Name(cluster=T18 {"BusIndex"=0, "clNetImpairTimeArray"=[]} ("clEvtReportArray"), "BusIndex"=w397, "clNetImpairTimeArray"=w394) -> (w392:T18)
            n166 = local read "QueName"() -> (w388:string)
            n167 = call "Enqueue.vi"("QueName"=w388, "Data"=w392, "Message"="NetImpairTime") -> ("Error"=w393:errorcluster[])  [unwired: 8 in]
          }
        }
      }
      event User Event {
        # "Enabled?"
        n168 = event-data() -> ("ModuleID"=w408:i32, "Data"=w407:variant)  [unwired: 1 in]
        n169 = case shown="True" TRUE {
          tunnel: w409 -> [w410 w412]
          tunnel: w408 -> [_ w421]
          tunnel: w407 -> [_ w419]
          tunnel: [_ w416] -> w406
          tunnel: [w410 w412] -> w404
          frame False {
          }
          frame True {
            # "Find Bus Index"
            n170 = for {
              tunnel: w412 -> [w426] mode=indexing
              tunnel: w421 -> [w424]
              tunnel: [w422] -> w420
              i -> [w422]
              stop <- w423 stop-if-true
              n171 = property class="Bus.lvclass"(reference=w426) -> ("Accessors:EventModuleID"=w425:i32)  [unwired: 1 in, 2 out]
              n172 = Equal?(x=w425, y=w424) -> (x = y?=w423:bool)
            }
            n173 = Variant To Data(type=T7 [] ("dblPktLoss"), Variant=w419) -> (data=w417:T7)  [unwired: 1 in, 1 out]
            n174 = Bundle By Name(cluster=T19 {"BusIndex"=0, "clNetPktLoss"=[]} ("clEvtReportArray"), "BusIndex"=w420, "clNetPktLoss"=w417) -> (w415:T19)
            n175 = local read "QueName"() -> (w411:string)
            n176 = call "Enqueue.vi"("QueName"=w411, "Data"=w415, "Message"="NetPktLoss") -> ("Error"=w416:errorcluster[])  [unwired: 8 in]
          }
        }
      }
      event User Event {
        # "Enabled?"
        n177 = event-data() -> ("ModuleID"=w431:i32, "Data"=w430:variant)  [unwired: 1 in]
        n178 = case shown="True" TRUE {
          tunnel: w432 -> [w433 w435]
          tunnel: w431 -> [_ w444]
          tunnel: w430 -> [_ w442]
          tunnel: [_ w439] -> w429
          tunnel: [w433 w435] -> w427
          frame False {
          }
          frame True {
            # "Find Bus Index"
            n179 = for {
              tunnel: w435 -> [w449] mode=indexing
              tunnel: w444 -> [w447]
              tunnel: [w445] -> w443
              i -> [w445]
              stop <- w446 stop-if-true
              n180 = property class="Bus.lvclass"(reference=w449) -> ("Accessors:EventModuleID"=w448:i32)  [unwired: 1 in, 2 out]
              n181 = Equal?(x=w448, y=w447) -> (x = y?=w446:bool)
            }
            n182 = Variant To Data(type=T8 [] ("ui32FlagImpairmentArray"), Variant=w442) -> (data=w440:T8)  [unwired: 1 in, 1 out]
            n183 = Bundle By Name(cluster=T20 {"BusIndex"=0, "FlagImpairArray"=[]} ("clEvtReportArray"), "BusIndex"=w443, "FlagImpairArray"=w440) -> (w438:T20)
            n184 = local read "QueName"() -> (w434:string)
            n185 = call "Enqueue.vi"("QueName"=w434, "Data"=w438, "Message"="FlagImpair") -> ("Error"=w439:errorcluster[])  [unwired: 8 in]
          }
        }
      }
      event "btnStop": Value Change {
        n186 = event-data() -> ()  [unwired: 1 in, 1 out]
        n187 = call "ObtainRequestEvents.vi"() -> ("Error"=w460:errorcluster[], "clRequestEvents"=w457:T9)  [unwired: 10 in]
        n188 = Unbundle By Name(w457) -> ("StopRequest"=w458:refnum<user-event>)
        n189 = Generate User Event(priority (normal)=usereventprio."high priority", user event=w458, event data cluster=T22 {"BusIndex"=0, "Data"=variant} ("event data")) -> (error out=w459:errorcluster)  [unwired: 1 in, 1 out]
        n190 = call <userlib>:"AddError.vi"("Severity"="Fatal" ("String"), "Priority"=u8 0, "ErrorArray"=w460, "error in (no error)"=w459) -> ("ErrorArray"=w456:errorcluster[], "error out"=w453:errorcluster)  [unwired: 6 in]
        n191 = call <vilib>:"Clear Errors.vi"("error in (no error)"=w453) -> ()  [unwired: 5 in, 2 out]
      }
    }
    n192 = local read "QueName"() -> (w231:string)
    n193 = call "EnqueError.vi"("QueName"=w231, "Error"=w236) -> ("Error"=w235:errorcluster[])  [unwired: 9 in]
  }
  n194 = Build Array (concatenate)(w25, w26) -> (→"ErrorArray":errorcluster[])
